vi "Pre Launch Init.vi"(11 "CS++IEFWerner in":refnum<class "CS++IEFWerner.lvclass">) -> (0 "error out":errorcluster, 3 "CS++IEFWerner out":refnum<class "CS++IEFWerner.lvclass">)   [LabVIEW 2015, in "CS++IEFWerner.lvlib" / "CS++IEFWerner.lvclass"]
doc: "(<B>Filename</B>: Actor Framework.lvlib:Actor.lvclass:Pre Launch Init.vi)\n\nDefines behavior that occurs after the Launch Actor method is invoked but before the actor's Actor Core method begins running.\n\nThe Pre Launch Init method is guaranteed to finish before the Launch Actor method returns to its caller and before the actor itself receives any messages. Any references that the Pre Launch Init method obtains are guaranteed to have the same lifetime as the actor itself. Any errors that the Pre Launch Init method returns will abort the launch.\n\nBy default, this method does nothing. A descendant class may override it to define behavior."
uses:
  CS++IEFWerner.lvclass
  CS++IEFWerner.lvclass/CS++IEFWerner.ctl
  CSPP_DeviceBase/CS++Motor/CS++Motor.lvclass
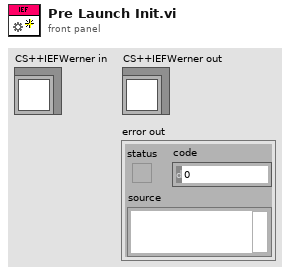
[diagram p1: front panel]
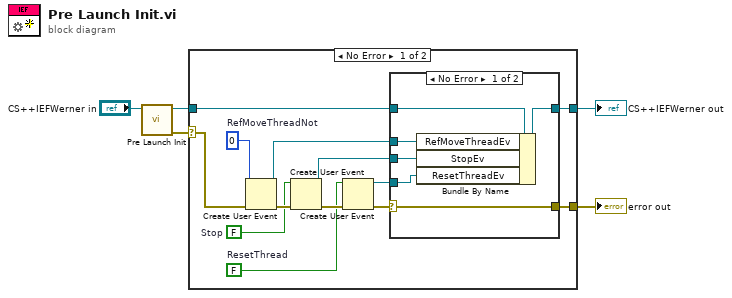
[diagram p0: block diagram]
diagram:
  n1 = call-parent "Pre Launch Init.vi"("CS++BaseActor in"="CS++IEFWerner in") -> ("error out"=w2:errorcluster, "CS++BaseActor out"=w3:refnum<class "CS++IEFWerner.lvclass">)  [unwired: 9 in]
  n2 = case shown="No Error" w2 {
    selector: w2 -> [w17 w27]
    tunnel: [w15 w28] -> w4
    tunnel: w3 -> [w14 w28]
    tunnel: [w16 w27] -> w1
    frame No Error {
      w7 = FALSE  # ResetThread
      w11 = FALSE  # Stop
      w18 = u16 0  # RefMoveThreadNot
      n3 = Create User Event(user event datatype=w18, error in=w17) -> (user event=w13:refnum<user-event>, error out=w12:errorcluster)
      n4 = Create User Event(user event datatype=w11, error in=w12) -> (user event=w10:refnum<user-event>, error out=w9:errorcluster)
      n5 = Create User Event(user event datatype=w7, error in=w9) -> (user event=w6:refnum<user-event>, error out=w8:errorcluster)
      n6 = case shown="No Error" w8 {
        selector: w8 -> [w24 w25]
        tunnel: [w24 w25] -> w16
        tunnel: [w22 w26] -> w15
        tunnel: w14 -> [w23 w26]
        tunnel: w13 -> [w21 _]
        tunnel: w10 -> [w20 _]
        tunnel: w6 -> [w19 _]
        frame No Error {
          n7 = Bundle By Name(cluster=w23, "RefMoveThreadEv"=w21, "StopEv"=w20, "ResetThreadEv"=w19) -> (w22:refnum<class "CS++IEFWerner.lvclass">)
        }
        frame Error {
        }
      }
    }
    frame Error {
    }
  }
  "error out" <- w1
  "CS++IEFWerner out" <- w4
